vi "saving.vi"(0 "file path (use dialog)":path=path "Z:/11 Setups/04 NOPA TA/01 Data/20211129/test/test", 1 "save type":bool[](array[boolean]), 2 "details":string[](array[string])=["Title", "Author", "Description"], 3 "signal mean":dbl[](array[numeric]), 5 "wavelength":dbl[](array[numeric]), 9 "time delays":dbl[][](array[numeric]), 11 "signal (accum.)":dbl[][](array[numeric]), 12 "raw data":dbl[][][](array[numeric]), 14 "reference mean":dbl[](array[numeric])) -> ()   [LabVIEW 2019]
uses:
  <vilib>/regexp/Match Regular Expression.xnode
panel:
  # "saving ..."
  # "transients"
  # "signal mean"
  # "reference mean"
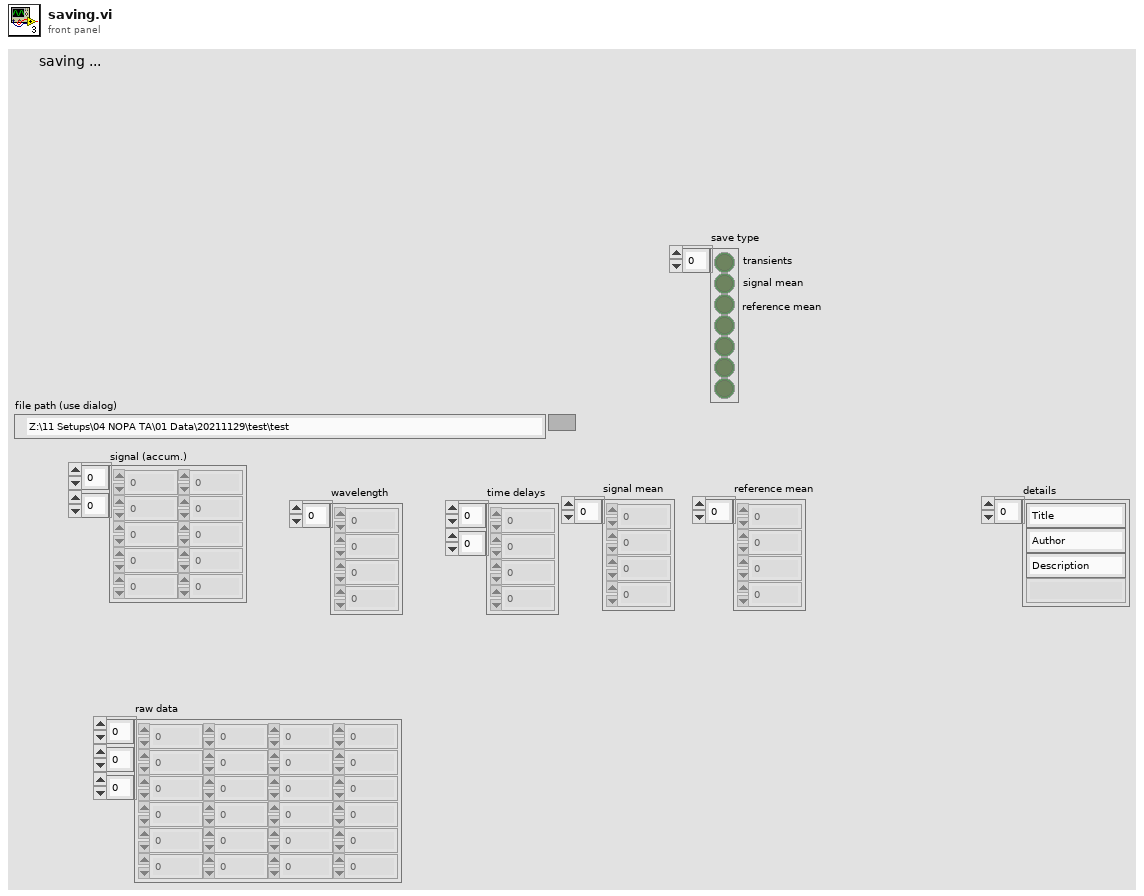
[diagram p1: front panel]
types:
  T1 = enum16{"open", "open or create", "create or replace", "create", "open (read-only)"}
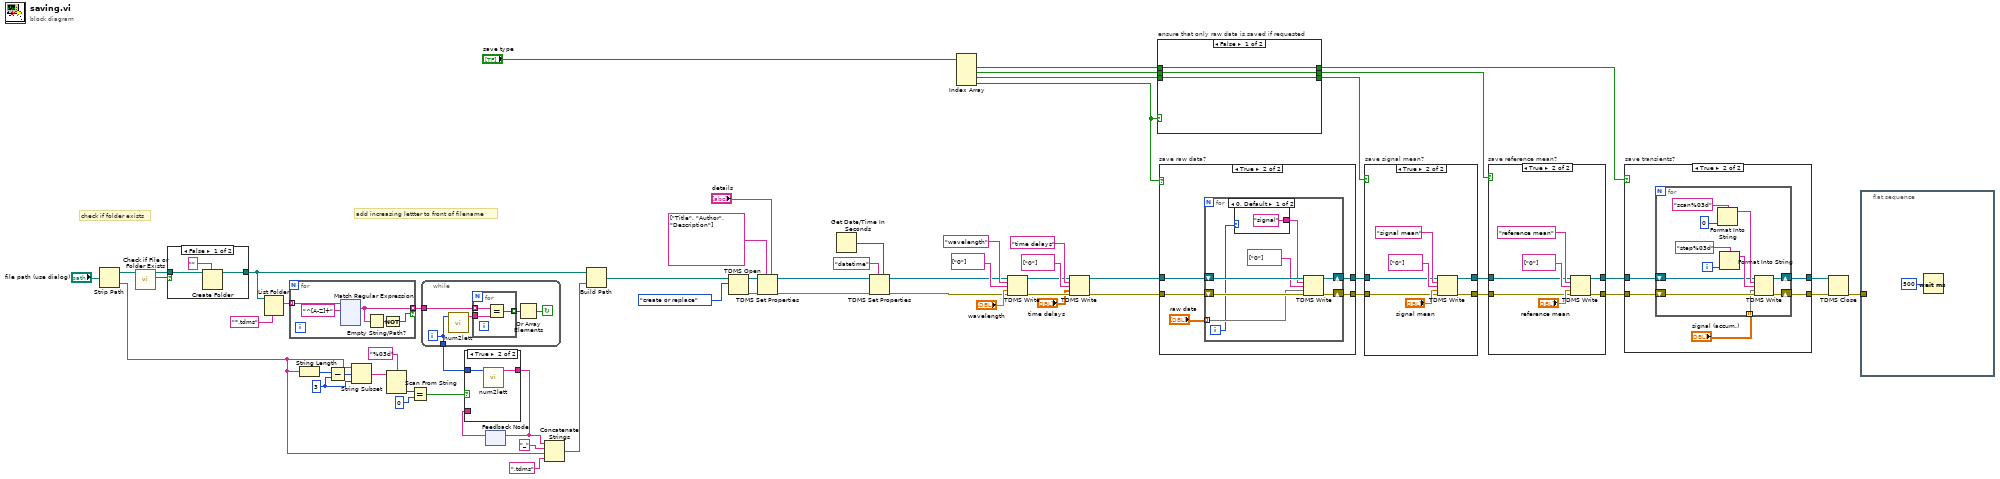
[diagram p0: block diagram]
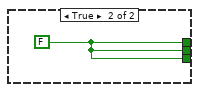
[diagram p2: hidden frame]
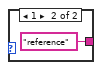
[diagram p4: hidden frame]
diagram:
  w31 = 3
  # "add increasing lettter to front of filename"
  # "check if folder exists"
  n1 = Strip Path(path="file path (use dialog)") -> (stripped path=w58:path, name=w23:string)
  n2 = call <vilib>:"Check if File or Folder Exists.vi"("path"=w58) -> ("file or folder exists?"=w61:bool, "dup path"=w60:path)  [unwired: 8 in, 1 out]
  n3 = case shown="False" w61 {
    tunnel: [w64 w66] -> w37
    tunnel: w60 -> [w63 w66]
    frame False {
      n4 = Create Folder(prompt (Create Folder)="", path (use dialog)=w63) -> (created path=w64:path)  [unwired: 1 in, 2 out]
    }
    frame True {
    }
  }
  n5 = List Folder(path=w37, pattern="*.tdms") -> (filenames=w36:string[])  [unwired: 2 in, 3 out]
  n6 = for {
    tunnel: w36 -> [w70] mode=indexing
    tunnel: [w69] -> w21 mode=indexing if=w67
    n7 = xnode "Match Regular Expression"("input string"=w70, "regular expression"="^[A-Z]+") -> ("whole match"=w69:string)  [unwired: 4 in, 4 out]
    n8 = Empty String/Path?(string/path=w69) -> (empty?=w68:bool)
    n9 = Not(x=w68) -> (.not. x?=w67:bool)
  }
  n10 = String Length(string=w23) -> (length=w33:i32)
  n11 = Subtract(x=w33, y=w31) -> (x-y=w32:i32)
  n12 = String Subset(string=w23, offset (0)=w32, length (rest)=w31) -> (substring=w30:string)
  n13 = Scan From String(format string="%03d", input string=w30) -> (output 1=w28:i32)  [unwired: 3 in, 3 out]
  n14 = Equal?(x=w28, y=0) -> (x = y?=w26:bool)
  n15 = while {
    tunnel: w21 -> [w190]
    tunnel: [w186] -> w20
    i -> [w186]
    stop <- w187 continue-if-true
    n16 = call "num2lett.vi"("Number"=w186) -> ("Letter"=w189:string)  [unwired: 10 in]
    n17 = for {
      tunnel: w190 -> [w192] mode=indexing
      tunnel: w189 -> [w193]
      tunnel: [w191] -> w188 mode=indexing
      n18 = Equal?(x=w192, y=w193) -> (x = y?=w191:bool)
    }
    n19 = Or Array Elements(Boolean array=w188) -> (logical OR=w187:bool)
  }
  n20 = feedback #1() -> (w24:string)  [unwired: 1 in]
  n21 = case shown="True" w26 {
    tunnel: [w194 w196] -> w22
    tunnel: w24 -> [w194 _]
    tunnel: w20 -> [_ w195]
    frame False {
    }
    frame True {
      n22 = call "num2lett.vi"("Number"=w195) -> ("Letter"=w196:string)  [unwired: 10 in]
    }
  }
  n23 = feedback-in #1(w22) -> ()
  n24 = Concatenate Strings(w22, "_" ("string"), w23, ".tdms" ("string")) -> (w34:string)
  n25 = Build Path(base path=w37, name or relative path=w34) -> (appended path=w39:path)
  n26 = TDMS Open(10:T1."create or replace" ("operation (0:open)"), 11:w39) -> (0:w49:errorcluster, 3:w56:refnum<k34>)  [unwired: 5 in]
  n27 = TDMS Set Properties(5:"details", 7:string[] ["Title", "Author", "Description"] ("property names"), 8:w49, 11:w56) -> (0:w5:errorcluster, 3:w6:refnum<k34>)  [unwired: 2 in, 2 out]
  n28 = Get Date/Time In Seconds() -> (seconds since 1Jan1904=w1:timestamp)
  n29 = TDMS Set Properties(5:w1, 7:"datetime", 8:w5, 11:w6) -> (0:w3:errorcluster, 3:w4:refnum<k34>)  [unwired: 2 in, 2 out]
  n30 = Index Array(array="save type") -> (element #1=w10:bool, element #2=w11:bool, element #3=w13:bool, element #4=w14:bool)  [unwired: 4 in]
  n31 = TDMS Write(0:w4, 5:"wavelength" ("group name in (Untitled)"), 7:string[] ["0"] ("channel name(s) in (Untitled)"), 9:"wavelength", 11:w3) -> (4:w50:refnum<k34>, 15:w48:errorcluster)  [unwired: 1 in, 2 out]
  n32 = TDMS Write(0:w50, 5:"time delays" ("group name in (Untitled)"), 7:string[] ["0"] ("channel name(s) in (Untitled)"), 9:"time delays", 11:w48) -> (4:w18:refnum<k34>, 15:w15:errorcluster)  [unwired: 1 in, 2 out]
  n33 = case "ensure that only raw data is saved if requested" shown="False" w14 {
    tunnel: w13 -> [w197 _]
    tunnel: [w197 w200] -> w12
    tunnel: w11 -> [w198 _]
    tunnel: w10 -> [w199 _]
    tunnel: [w199 w200] -> w9
    tunnel: [w198 w200] -> w8
    frame False {
    }
    frame True {
      w200 = FALSE
    }
  }
  n34 = case "save raw data?" shown="True" w14 {
    tunnel: w18 -> [w202 w207]
    tunnel: [w202 w204] -> w17
    tunnel: [w201 w205] -> w16
    tunnel: w15 -> [w201 w206]
    frame False {
    }
    frame True {
      n35 = for {
        shift-right: [w213] -> w205
        shift-left: w206 -> [w214]
        shift-right: [w212] -> w204
        shift-left: w207 -> [w215]
        tunnel: "raw data" -> [w211] mode=indexing
        i -> [w208]
        n36 = case shown="0, Default" w208 {
          tunnel: ["signal" ("group name in (Untitled)") "reference" ("group name in (Untitled)")] -> w210
          frame 0, Default {
          }
          frame 1 {
          }
        }
        n37 = TDMS Write(0:w215, 5:w210, 7:string[] ["0"] ("channel name(s) in (Untitled)"), 9:w211, 11:w214) -> (4:w212:refnum<k34>, 15:w213:errorcluster)  [unwired: 1 in, 2 out]
      }
    }
  }
  n38 = case "save signal mean?" shown="True" w12 {
    tunnel: w17 -> [w219 w223]
    tunnel: w16 -> [w218 w222]
    tunnel: [w219 w221] -> w43
    tunnel: [w218 w220] -> w42
    frame False {
    }
    frame True {
      n39 = TDMS Write(0:w223, 5:"signal mean" ("group name in (Untitled)"), 7:string[] ["0"] ("channel name(s) in (Untitled)"), 9:"signal mean", 11:w222) -> (4:w221:refnum<k34>, 15:w220:errorcluster)  [unwired: 1 in, 2 out]
    }
  }
  n40 = case "save reference mean?" shown="True" w8 {
    tunnel: w43 -> [w228 w232]
    tunnel: w42 -> [w227 w231]
    tunnel: [w227 w230] -> w41
    tunnel: [w228 w229] -> w40
    frame False {
      # "save reference mean"
    }
    frame True {
      n41 = TDMS Write(0:w232, 5:"reference mean" ("group name in (Untitled)"), 7:string[] ["0"] ("channel name(s) in (Untitled)"), 9:"reference mean", 11:w231) -> (4:w229:refnum<k34>, 15:w230:errorcluster)  [unwired: 1 in, 2 out]
    }
  }
  n42 = case "save transients?" shown="True" w9 {
    tunnel: w40 -> [w237 w242]
    tunnel: w41 -> [w236 w241]
    tunnel: [w237 w240] -> w47
    tunnel: [w236 w239] -> w46
    frame False {
      # "save transient"
    }
    frame True {
      # "save transients"
      n43 = for {
        tunnel: "signal (accum.)" -> [w243] mode=indexing
        shift-right: [w246] -> w240
        shift-left: w242 -> [w248]
        shift-right: [w245] -> w239
        shift-left: w241 -> [w247]
        i -> [w244]
        n44 = Format Into String(format string="scan%03d" ("initial string"), 0) -> (resulting string=w253:string)  [unwired: 2 in, 1 out]
        n45 = Format Into String(format string="step%03d" ("initial string"), w244) -> (resulting string=w249:string)  [unwired: 2 in, 1 out]
        n46 = TDMS Write(0:w248, 5:w253, 7:w249, 9:w243, 11:w247) -> (4:w246:refnum<k34>, 15:w245:errorcluster)  [unwired: 1 in, 2 out]
      }
    }
  }
  n47 = TDMS Close(8:w46, 11:w47) -> (0:w25:errorcluster)  [unwired: 1 out]
  n48 = flat-sequence {
    tunnel: w25 -> [_]
    frame #0 {
      n49 = Wait (ms)(milliseconds to wait=u32 500) -> ()  [unwired: 1 out]
    }
  }
